vi "On.vi"(8 "error in (no error)":errorcluster, 11 "reference in":refnum<class "Light.lvclass">) -> (0 "error out":errorcluster, 3 "reference out":refnum<class "Light.lvclass">)   [LabVIEW 2012, in "Light.lvclass"]
uses:
  Light.lvclass
  <userlib>/_LabVIEWCommon/LcDialogs/LcDialog_AutoSizeDialog_Font.ctl
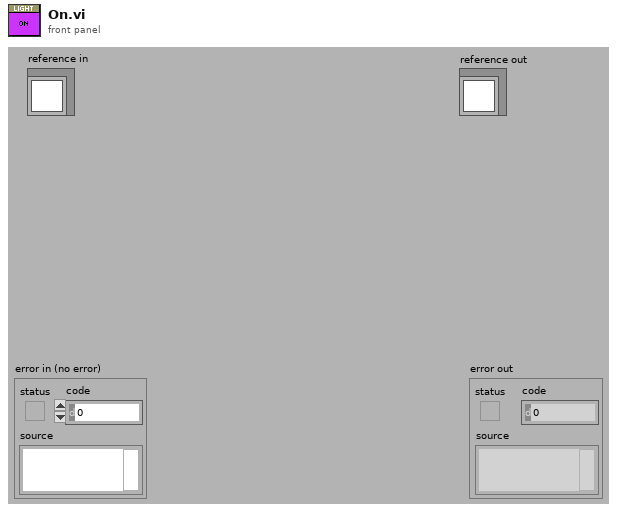
[diagram p1: front panel]
types:
  T1 = typedef "LcDialog_AutoSizeDialog_Font.ctl" = cluster{"Size":u32, "Bold":bool, "Color":u32}
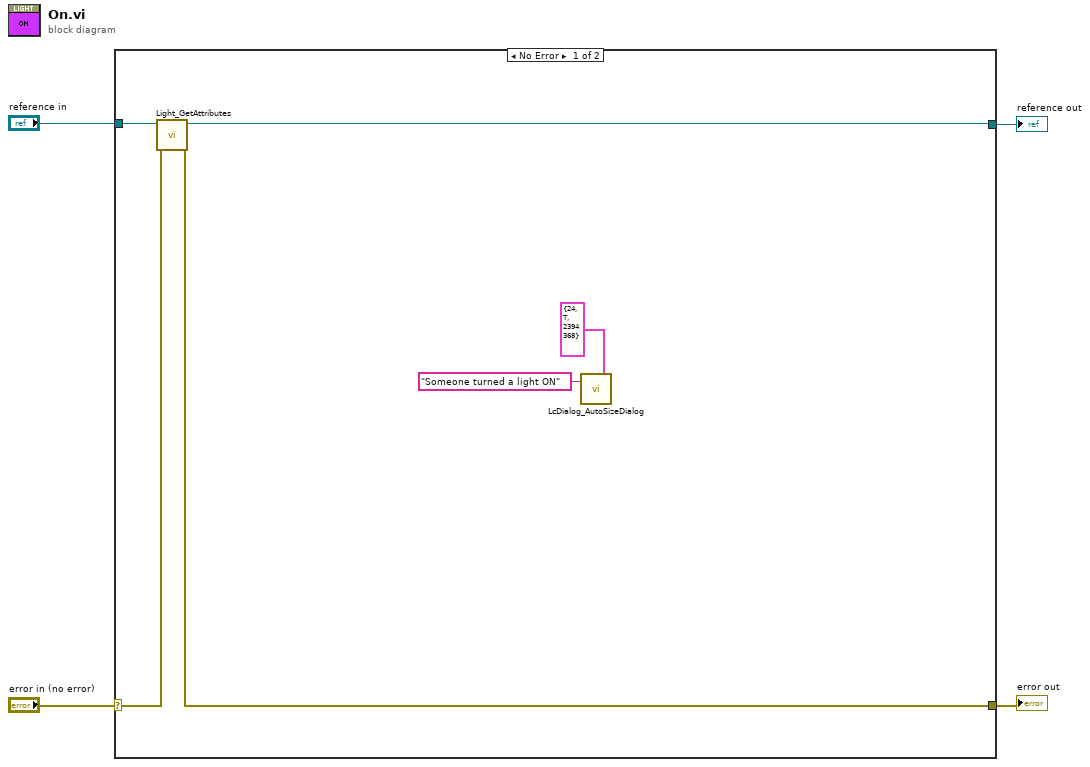
[diagram p0: block diagram]
diagram:
  n1 = case shown="No Error" "error in (no error)" {
    selector: "error in (no error)" -> [w9 w12]
    tunnel: [w7 w12] -> w3
    tunnel: [w8 w11] -> w1
    tunnel: "reference in" -> [w10 w11]
    frame No Error {
      n2 = call "Light_GetAttributes.vi"("error in (no error)"=w9, "reference in"=w10) -> ("error out"=w7:errorcluster, "reference out"=w8:refnum<class "Light.lvclass">)  [unwired: 6 in, 2 out]
      n3 = call <userlib>:"LcDialog_AutoSizeDialog.vi"("TextIn"="Someone turned a light ON", "FontSettings"=T1 {"Size"=24, "Bold"=TRUE, "Color"=2394368}) -> ()  [unwired: 13 in, 5 out]
    }
    frame Error {
    }
  }
  "error out" <- w3
  "reference out" <- w1
